vi "Operator ID.vi"(0 "Enable":bool=TRUE, 1 "Strings []":string[](array[string]), 5 "error in (no error)":errorcluster) -> (14 "Temp sensor out":T1, 15 "Varaint Selection out":string(combo), 17 "Operator ID":i32, 18 "OK":bool, 19 "error out":errorcluster)   [LabVIEW 2021]
doc: "Displays a standard dialog box that prompts users to enter information, such as a user name and password.\n--------------------\n\nThis Express VI is configured as follows:\n\nMessage to Display to the User:\nThe inputs are: \nText Entry Box: Operator ID"
uses:
  controls/Control 1.ctl
panel:
  in  "Temp sensor":T1
  in  "Variant Selection":string(combo)
  in  "Operator ID":i32
  in  "Cancel":bool
  in  "OK2":bool
  in  "OK1":bool
  # "Enter operator ID and press OK"
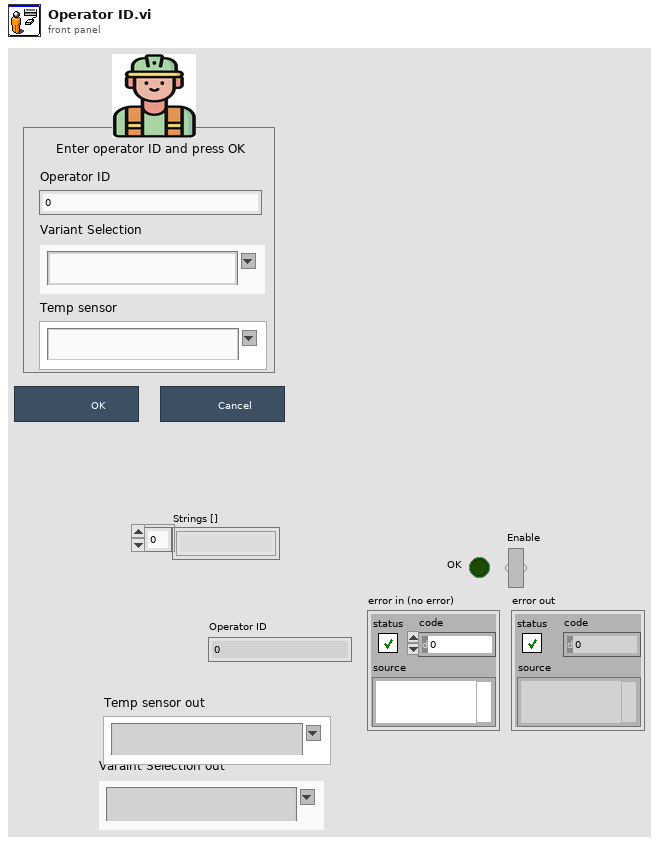
[diagram p1: front panel]
types:
  T1 = typedef "Control 1.ctl" = string
  T2 = cluster{"Input Name":string, "Input Data Type":i32}[]
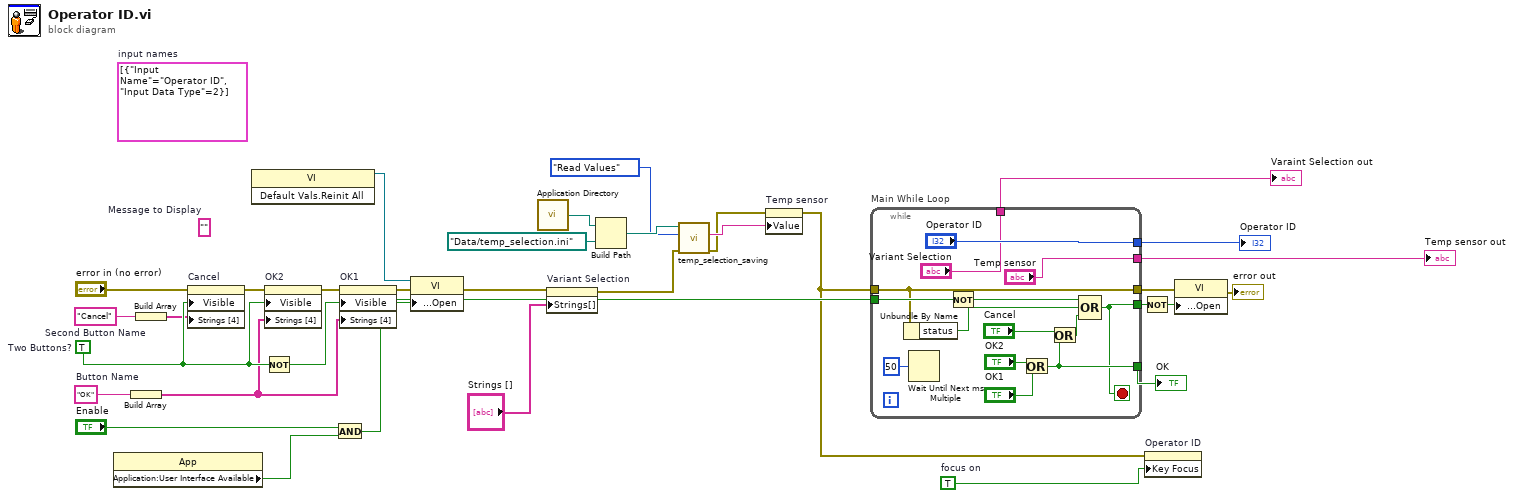
[diagram p0: block diagram]
diagram:
  w13 = TRUE  # focus on
  (unwired) T2 [{"Input Name"="Operator ID", "Input Data Type"=2}]  # input names
  w25 = "Cancel"  # Second Button Name
  w23 = "OK"  # Button Name
  (unwired) ""  # Message to Display
  w33 = TRUE  # Two Buttons?
  n1 = property class="App"() -> ("Application:User Interface Available"=w16:bool)  [unwired: 2 in, 2 out]
  n2 = Build Array(w23) -> (w24:string[])
  n3 = Build Array(w25) -> (w26:string[])
  n4 = property on="Cancel" class="Bool"(error in="error in (no error)", "Visible"=w33, "Strings [4]"=w26) -> (error out=w30:errorcluster)  [unwired: 1 in, 1 out]
  n5 = invoke class="VI" method="Default Vals.Reinit All"() -> (reference out=w15:refnum<vi>)  [unwired: 3 in, 2 out]
  n6 = Not(x=w33) -> (.not. x?=w31:bool)
  n7 = property on="OK2" class="Bool"(error in=w30, "Visible"=w33, "Strings [4]"=w24) -> (error out=w29:errorcluster)  [unwired: 1 in, 1 out]
  n8 = And(x="Enable", y=w16) -> (x .and. y?=w17:bool)
  n9 = property on="OK1" class="Bool"(error in=w29, "Visible"=w31, "Strings [4]"=w24) -> (error out=w22:errorcluster)  [unwired: 1 in, 1 out]
  n10 = property class="VI"(reference=w15, error in=w22, "Front Panel Window:Open"=w17) -> (error out=w10:errorcluster)  [unwired: 1 out]
  n11 = call <vilib>:"Application Directory.vi"() -> ("Application Directory"=w6:path)
  n12 = property on="Variant Selection" class="CmbBox"(error in=w10, "Strings[]"="Strings []") -> (error out=w8:errorcluster)  [unwired: 1 in, 1 out]
  n13 = Build Path(base path=w6, name or relative path=path "Data/temp_selection.ini") -> (appended path=w7:path)
  n14 = call "temp_selection_saving.vi"("error in (no error)"=w8, "Enum"=enum16{"Write", "Read Values"}."Read Values", "configuration file path"=w7) -> ("error out"=w2:errorcluster, "selection_temp"=w3:string)  [unwired: 6 in, 1 out]
  n15 = property on="Temp sensor" class="CmbBox (strict)"(error in=w2, "Value"=w3) -> (error out=w1:errorcluster)  [unwired: 1 in, 1 out]
  n16 = while "Main While Loop" {
    tunnel: [w44] -> w32
    tunnel: w17 -> [w42]
    tunnel: [w40] -> w27
    tunnel: w1 -> [w39]
    tunnel: [w39] -> w20
    tunnel: ["Operator ID"] -> w14
    tunnel: ["Variant Selection"] -> w12
    tunnel: ["Temp sensor"] -> w11
    stop <- w40 stop-if-true
    n17 = Unbundle By Name(w39) -> ("status"=w37:bool)
    n18 = Wait Until Next ms Multiple(millisecond multiple=u32 50) -> ()  [unwired: 1 out]
    n19 = Not(x=w42) -> (.not. x?=w41:bool)
    n20 = Or(x="OK2", y="OK1") -> (x .or. y?=w44:bool)
    n21 = Or(x="Cancel", y=w44) -> (x .or. y?=w38:bool)
    n22 = Compound Arithmetic op=OR(w41, w37, w38) -> (w40:bool)
  }
  "OK" <- w32
  "Operator ID" <- w14
  "Varaint Selection out" <- w12
  "Temp sensor out" <- w11
  n23 = Not(x=w27) -> (.not. x?=w28:bool)
  n24 = property on="Operator ID" class="DigNum (strict)"(error in=w1, "Key Focus"=w13) -> ()  [unwired: 1 in, 2 out]
  n25 = property class="VI"(error in=w20, "Front Panel Window:Open"=w28) -> (error out=→"error out":errorcluster)  [unwired: 1 in, 1 out]
